vi "Main.vi"(7 "sweep rate, /min":dbl=0.2, 8 "sweep to:":dbl=-0.5, 9 "sweep":T6(radio)=enum."time_sweep") -> ()   [LabVIEW 2017] (continued)
                  n2525 = case shown="False" w3354 {
                    tunnel: w3355 -> [w3357 w3370]
                    tunnel: [w3357 w3369] -> w3356
                    frame False {
                      # "we are not measuring 2182A 4 channel 2 (2182A_4_ch2)"
                    }
                    frame True {
                      # "switching to channel 2 and then\nback to channel 1"
                      # "we are  measuring 2182A 4 channel 2 (2182A_4_ch2)"
                      n2526 = local read "2182A 4 addr"() -> (w3364:u8)
                      n2527 = Number To Decimal String(number=w3364) -> (decimal integer string=w3359:string)  [unwired: 1 in]
                      n2528 = GPIB Write(0:w3359, 1:":SENSe:CHAN 2") -> (6:w3361:errorcluster)  [unwired: 3 in, 1 out]
                      n2529 = GPIB Write(0:w3359, 1:":SENSe:DATA:FRES?", 3:w3361) -> (6:w3368:errorcluster)  [unwired: 2 in, 1 out]
                      n2530 = GPIB Read(0:w3359, 1:200, 3:w3368) -> (5:w3363:string, 7:w3360:errorcluster)  [unwired: 2 in, 1 out]
                      n2531 = GPIB Write(0:w3359, 1:":SENSe:CHAN 1", 3:w3360) -> ()  [unwired: 2 in, 2 out]
                      n2532 = Fract/Exp String To Number(string=w3363) -> (number=w3366:dbl)  [unwired: 3 in, 1 out]
                      n2533 = Build Array (concatenate)(w3370, w3366) -> (w3369:dbl[])
                    }
                  }
                  n2534 = property on="data" class="Arr (strict)"("Value"=w3356) -> ()  [unwired: 2 in, 2 out]
                }
                frame #34 {
                  # "check if voltage on\nKeithley 2636A smua\nis to be measured"
                  n2535 = local read "2636A smua meas v"() -> (w3371:bool)
                  n2536 = property on="data" class="Arr (strict)"() -> ("Value"=w3372:dbl[])  [unwired: 2 in, 2 out]
                  n2537 = case shown="True" w3371 {
                    tunnel: w3372 -> [w3374 w3380]
                    tunnel: [w3374 w3379] -> w3373
                    frame False {
                      # "we are not measuring voltage on 2636A smua (2636A_smua_v)"
                    }
                    frame True {
                      # "we are  measuring voltage on 2636A smua (2636A_smua_v)"
                      n2538 = local read "2336A addr"() -> (w3375:refnum<visa-resource-name>)
                      n2539 = call "SinglePointMeasurement.vi"("Measure"=Measure."Voltage", "Channel"=Channel."a", "VISA resource name 2"=w3375) -> ("Measuremet"=w3377:dbl)  [unwired: 3 in, 4 out]
                      n2540 = Build Array (concatenate)(w3380, w3377) -> (w3379:dbl[])
                    }
                  }
                  n2541 = property on="data" class="Arr (strict)"("Value"=w3373) -> ()  [unwired: 2 in, 2 out]
                }
                frame #35 {
                  # "check if current on\nKeithley 2636A smua\nis to be measured"
                  n2542 = local read "2636A smua meas i"() -> (w3381:bool)
                  n2543 = property on="data" class="Arr (strict)"() -> ("Value"=w3382:dbl[])  [unwired: 2 in, 2 out]
                  n2544 = case shown="True" w3381 {
                    tunnel: w3382 -> [w3384 w3387]
                    tunnel: [w3384 w3386] -> w3383
                    frame False {
                      # "we are not measuring current on 2636A smua (2636A_smua_i)"
                    }
                    frame True {
                      # "we are  measuring current on 2636A smua (2636A_smua_i)"
                      n2545 = stacked-sequence {
                        tunnel: [_ w3396] -> w3385
                        frame #0 {
                          n2546 = local read "auto\nrange A"() -> (w3391:bool)
                          n2547 = local read "2336A addr"() -> (w3394:refnum<visa-resource-name>)
                          n2548 = Select(t="smua.AUTORANGE_ON", s=w3391, f="smua.AUTORANGE_OFF") -> (s? t:f=w3389:string)
                          n2549 = Concatenate Strings("smua.measure.autorangei = ", w3389) -> (w3388:string)
                          n2550 = VISA Write(VISA resource name=w3394, write buffer=w3388) -> ()  [unwired: 1 in, 3 out]
                        }
                        frame #1 {
                          n2551 = local read "2336A addr"() -> (w3398:refnum<visa-resource-name>)
                          n2552 = call "SinglePointMeasurement.vi"("Measure"=Measure."Current", "Channel"=Channel."a", "VISA resource name 2"=w3398) -> ("Measuremet"=w3396:dbl)  [unwired: 3 in, 4 out]
                        }
                      }
                      n2553 = Build Array (concatenate)(w3387, w3385) -> (w3386:dbl[])
                    }
                  }
                  n2554 = property on="data" class="Arr (strict)"("Value"=w3383) -> ()  [unwired: 2 in, 2 out]
                }
                frame #36 {
                  # "check if voltage on\nKeithley 2636A smub\nis to be measured"
                  n2555 = local read "2636A smub meas v"() -> (w3399:bool)
                  n2556 = property on="data" class="Arr (strict)"() -> ("Value"=w3400:dbl[])  [unwired: 2 in, 2 out]
                  n2557 = case shown="True" w3399 {
                    tunnel: w3400 -> [w3402 w3408]
                    tunnel: [w3402 w3407] -> w3401
                    frame False {
                      # "we are not measuring voltage on 2636A smub (2636A_smub_v)"
                    }
                    frame True {
                      # "we are  measuring voltage on 2636A smub (2636A_smub_v)"
                      n2558 = local read "2336A addr"() -> (w3406:refnum<visa-resource-name>)
                      n2559 = call "SinglePointMeasurement.vi"("Measure"=Measure."Voltage", "Channel"=Channel."b", "VISA resource name 2"=w3406) -> ("Measuremet"=w3404:dbl)  [unwired: 3 in, 4 out]
                      n2560 = Build Array (concatenate)(w3408, w3404) -> (w3407:dbl[])
                    }
                  }
                  n2561 = property on="data" class="Arr (strict)"("Value"=w3401) -> ()  [unwired: 2 in, 2 out]
                }
                frame #37 {
                  # "check if current on\nKeithley 2636A smub\nis to be measured"
                  n2562 = local read "2636A smub meas i"() -> (w3409:bool)
                  n2563 = property on="data" class="Arr (strict)"() -> ("Value"=w3410:dbl[])  [unwired: 2 in, 2 out]
                  n2564 = case shown="True" w3409 {
                    tunnel: w3410 -> [w3412 w3415]
                    tunnel: [w3412 w3414] -> w3411
                    frame False {
                      # "we are not measuring current on 2636A smub (2636A_smub_i)"
                    }
                    frame True {
                      # "we are  measuring current on 2636A smub (2636A_smub_i)"
                      n2565 = stacked-sequence {
                        tunnel: [_ w3424] -> w3413
                        frame #0 {
                          n2566 = local read "auto\nrange B"() -> (w3419:bool)
                          n2567 = local read "2336A addr"() -> (w3422:refnum<visa-resource-name>)
                          n2568 = Select(t="smub.AUTORANGE_ON", s=w3419, f="smub.AUTORANGE_OFF") -> (s? t:f=w3417:string)
                          n2569 = Concatenate Strings("smub.measure.autorangei = ", w3417) -> (w3416:string)
                          n2570 = VISA Write(VISA resource name=w3422, write buffer=w3416) -> ()  [unwired: 1 in, 3 out]
                        }
                        frame #1 {
                          n2571 = local read "2336A addr"() -> (w3426:refnum<visa-resource-name>)
                          n2572 = call "SinglePointMeasurement.vi"("Measure"=Measure."Current", "Channel"=Channel."b", "VISA resource name 2"=w3426) -> ("Measuremet"=w3424:dbl)  [unwired: 3 in, 4 out]
                        }
                      }
                      n2573 = Build Array (concatenate)(w3415, w3413) -> (w3414:dbl[])
                    }
                  }
                  n2574 = property on="data" class="Arr (strict)"("Value"=w3411) -> ()  [unwired: 2 in, 2 out]
                }
                frame #38 {
                  # "check if time\nis to be measured"
                  n2575 = property on="data" class="Arr (strict)"() -> ("Value"=w3429:dbl[])  [unwired: 2 in, 2 out]
                  n2576 = local read "measure time"() -> (w3428:bool)
                  n2577 = case shown="True" w3428 {
                    tunnel: w3429 -> [w3431 w3437]
                    tunnel: [w3431 w3436] -> w3430
                    tunnel: w3427 -> [_ w3434]
                    frame False {
                      # "we are not measuring time"
                    }
                    frame True {
                      # "seconds from the beginning of month"
                      # "we are  measuring time"
                      n2578 = call "timeInSeconds.vi"() -> ("Numeric"=w3435:dbl, "current time"=w3432:timestamp)  [unwired: 2 in]
                      n2579 = property on="current time" class="AbsTime (strict)"("Value"=w3432) -> ()  [unwired: 2 in, 2 out]
                      n2580 = Subtract(x=w3435, y=w3434) -> (x-y=w3433:dbl)
                      n2581 = Build Array (concatenate)(w3437, w3433) -> (w3436:dbl[])
                    }
                  }
                  n2582 = property on="data" class="Arr (strict)"("Value"=w3430) -> ()  [unwired: 2 in, 2 out]
                }
                frame #39 {
                  n2583 = local read "iPS_MagnetField"() -> (w3438:bool)
                  n2584 = property on="data" class="Arr (strict)"() -> ("Value"=w3439:dbl[])  [unwired: 2 in, 2 out]
                  n2585 = case shown="True" w3438 {
                    tunnel: w3439 -> [w3441 w3446]
                    tunnel: [w3441 w3445] -> w3440
                    frame False {
                      # "we are not Measuring magnetic field on IPS120-0"
                    }
                    frame True {
                      # "Measure magnetic field on Teslatron_iPS_Field"
                      n2586 = local read "iPS_addr_sweep"() -> (w3444:refnum<visa-resource-name>)
                      n2587 = call "iPSread.vi"("iPSreadCtrl"=iPSreadCtrl."MagnetField", "VISA resource name"=w3444) -> ("number"=w3443:dbl)  [unwired: 6 in, 3 out]
                      n2588 = Build Array (concatenate)(w3446, w3443) -> (w3445:dbl[])
                    }
                  }
                  n2589 = property on="data" class="Arr (strict)"("Value"=w3440) -> ()  [unwired: 2 in, 2 out]
                }
                frame #40 {
                  n2590 = property on="data" class="Arr (strict)"() -> ("Value"=w3448:dbl[])  [unwired: 2 in, 2 out]
                  n2591 = property on="Magnet_T" class="Bool (strict)"() -> ("Value"=w3447:bool)  [unwired: 2 in, 2 out]
                  n2592 = case shown="True" w3447 {
                    tunnel: w3448 -> [w3450 w3455]
                    tunnel: [w3450 w3454] -> w3449
                    frame False {
                      # "we are not Measuring magnetic field on IPS120-0"
                    }
                    frame True {
                      # "Measure magnetic_T on Teslatron"
                      n2593 = local read "iPS_addr_sweep"() -> (w3453:refnum<visa-resource-name>)
                      n2594 = call "iPSread.vi"("iPSreadCtrl"=iPSreadCtrl."Magnet Temp", "VISA resource name"=w3453) -> ("number"=w3452:dbl)  [unwired: 6 in, 3 out]
                      n2595 = Build Array (concatenate)(w3455, w3452) -> (w3454:dbl[])
                    }
                  }
                  n2596 = property on="data" class="Arr (strict)"("Value"=w3449) -> ()  [unwired: 2 in, 2 out]
                }
                frame #41 {
                  n2597 = property on="data" class="Arr (strict)"() -> ("Value"=w3457:dbl[])  [unwired: 2 in, 2 out]
                  n2598 = property on="SH_T" class="Bool (strict)"() -> ("Value"=w3456:bool)  [unwired: 2 in, 2 out]
                  n2599 = case shown="True" w3456 {
                    tunnel: w3457 -> [w3459 w3464]
                    tunnel: [w3459 w3463] -> w3458
                    frame False {
                      # "we are not Measuring magnetic field on IPS120-0"
                    }
                    frame True {
                      # "Measure  SH_T on Teslatron"
                      n2600 = local read "iPS_addr_sweep"() -> (w3462:refnum<visa-resource-name>)
                      n2601 = call "iPSread.vi"("iPSreadCtrl"=iPSreadCtrl."Switch Heater Temp", "VISA resource name"=w3462) -> ("number"=w3461:dbl)  [unwired: 6 in, 3 out]
                      n2602 = Build Array (concatenate)(w3464, w3461) -> (w3463:dbl[])
                    }
                  }
                  n2603 = property on="data" class="Arr (strict)"("Value"=w3458) -> ()  [unwired: 2 in, 2 out]
                }
                frame #42 {
                  # "check if current \non 2461 SouceMeter\nis to be measured"
                  n2604 = property on="data" class="Arr (strict)"() -> ("Value"=w3466:dbl[])  [unwired: 2 in, 2 out]
                  n2605 = property on="iTC_Sample_T" class="Bool (strict)"() -> ("Value"=w3465:bool)  [unwired: 2 in, 2 out]
                  n2606 = case shown="True" w3465 {
                    tunnel: w3466 -> [w3468 w3473]
                    tunnel: [w3468 w3472] -> w3467
                    frame False {
                      # "we are not measuring 2461, voltage (2461_meas_v)"
                    }
                    frame True {
                      # "we are  measuring 2461, voltage (2461_meas_v)"
                      n2607 = property on="iTC_addr_sweep" class="VISAName"() -> ("Value"=w3471:refnum<visa-resource-name>)  [unwired: 2 in, 2 out]
                      n2608 = call "iTCread.vi"("VISA resource name"=w3471, "iTCreadCtrl"=iTCreadCtrl."Sample Temp") -> ("number"=w3469:dbl)  [unwired: 5 in, 3 out]
                      n2609 = Build Array (concatenate)(w3473, w3469) -> (w3472:dbl[])
                    }
                  }
                  n2610 = property on="data" class="Arr (strict)"("Value"=w3467) -> ()  [unwired: 2 in, 2 out]
                }
                frame #43 {
                  # "check if current \non 2461 SouceMeter\nis to be measured"
                  n2611 = property on="data" class="Arr (strict)"() -> ("Value"=w3475:dbl[])  [unwired: 2 in, 2 out]
                  n2612 = property on="VTI_T" class="Bool (strict)"() -> ("Value"=w3474:bool)  [unwired: 2 in, 2 out]
                  n2613 = case shown="True" w3474 {
                    tunnel: w3475 -> [w3477 w3482]
                    tunnel: [w3477 w3481] -> w3476
                    frame False {
                      # "we are not measuring 2461, voltage (2461_meas_v)"
                    }
                    frame True {
                      # "we are  measuring 2461, voltage (2461_meas_v)"
                      n2614 = property on="iTC_addr_sweep" class="VISAName"() -> ("Value"=w3480:refnum<visa-resource-name>)  [unwired: 2 in, 2 out]
                      n2615 = call "iTCread.vi"("VISA resource name"=w3480, "iTCreadCtrl"=iTCreadCtrl."VTI Temp") -> ("number"=w3478:dbl)  [unwired: 5 in, 3 out]
                      n2616 = Build Array (concatenate)(w3482, w3478) -> (w3481:dbl[])
                    }
                  }
                  n2617 = property on="data" class="Arr (strict)"("Value"=w3476) -> ()  [unwired: 2 in, 2 out]
                }
                frame #44 {
                  # "check if current \non 2461 SouceMeter\nis to be measured"
                  n2618 = property on="data" class="Arr (strict)"() -> ("Value"=w3484:dbl[])  [unwired: 2 in, 2 out]
                  n2619 = property on="PT1_T" class="Bool (strict)"() -> ("Value"=w3483:bool)  [unwired: 2 in, 2 out]
                  n2620 = case shown="True" w3483 {
                    tunnel: w3484 -> [w3486 w3491]
                    tunnel: [w3486 w3490] -> w3485
                    frame False {
                      # "we are not measuring 2461, voltage (2461_meas_v)"
                    }
                    frame True {
                      # "we are  measuring 2461, voltage (2461_meas_v)"
                      n2621 = property on="iTC_addr_sweep" class="VISAName"() -> ("Value"=w3489:refnum<visa-resource-name>)  [unwired: 2 in, 2 out]
                      n2622 = call "iTCread.vi"("VISA resource name"=w3489, "iTCreadCtrl"=iTCreadCtrl."PT1 Temp") -> ("number"=w3487:dbl)  [unwired: 5 in, 3 out]
                      n2623 = Build Array (concatenate)(w3491, w3487) -> (w3490:dbl[])
                    }
                  }
                  n2624 = property on="data" class="Arr (strict)"("Value"=w3485) -> ()  [unwired: 2 in, 2 out]
                }
                frame #45 {
                  # "check if current \non 2461 SouceMeter\nis to be measured"
                  n2625 = property on="data" class="Arr (strict)"() -> ("Value"=w3493:dbl[])  [unwired: 2 in, 2 out]
                  n2626 = property on="PT2_T" class="Bool (strict)"() -> ("Value"=w3492:bool)  [unwired: 2 in, 2 out]
                  n2627 = case shown="True" w3492 {
                    tunnel: w3493 -> [w3495 w3500]
                    tunnel: [w3495 w3499] -> w3494
                    frame False {
                      # "we are not measuring 2461, voltage (2461_meas_v)"
                    }
                    frame True {
                      # "we are  measuring 2461, voltage (2461_meas_v)"
                      n2628 = property on="iTC_addr_sweep" class="VISAName"() -> ("Value"=w3498:refnum<visa-resource-name>)  [unwired: 2 in, 2 out]
                      n2629 = call "iTCread.vi"("VISA resource name"=w3498, "iTCreadCtrl"=iTCreadCtrl."PT2 Temp") -> ("number"=w3496:dbl)  [unwired: 5 in, 3 out]
                      n2630 = Build Array (concatenate)(w3500, w3496) -> (w3499:dbl[])
                    }
                  }
                  n2631 = property on="data" class="Arr (strict)"("Value"=w3494) -> ()  [unwired: 2 in, 2 out]
                }
                frame #46 {
                  # "check if current \non 2461 SouceMeter\nis to be measured"
                  n2632 = property on="data" class="Arr (strict)"() -> ("Value"=w3502:dbl[])  [unwired: 2 in, 2 out]
                  n2633 = property on="VTI_P" class="Bool (strict)"() -> ("Value"=w3501:bool)  [unwired: 2 in, 2 out]
                  n2634 = case shown="True" w3501 {
                    tunnel: w3502 -> [w3504 w3509]
                    tunnel: [w3504 w3508] -> w3503
                    frame False {
                      # "we are not measuring 2461, voltage (2461_meas_v)"
                    }
                    frame True {
                      # "we are  measuring 2461, voltage (2461_meas_v)"
                      n2635 = property on="iTC_addr_sweep" class="VISAName"() -> ("Value"=w3507:refnum<visa-resource-name>)  [unwired: 2 in, 2 out]
                      n2636 = call "iTCread.vi"("VISA resource name"=w3507, "iTCreadCtrl"=iTCreadCtrl."VTI Pressure") -> ("number"=w3505:dbl)  [unwired: 5 in, 3 out]
                      n2637 = Build Array (concatenate)(w3509, w3505) -> (w3508:dbl[])
                    }
                  }
                  n2638 = property on="data" class="Arr (strict)"("Value"=w3503) -> ()  [unwired: 2 in, 2 out]
                }
                frame #47 {
                  # "check if current \non 2461 SouceMeter\nis to be measured"
                  n2639 = property on="2461_meas_v" class="Bool (strict)"() -> ("Value"=w3510:bool)  [unwired: 2 in, 2 out]
                  n2640 = property on="data" class="Arr (strict)"() -> ("Value"=w3511:dbl[])  [unwired: 2 in, 2 out]
                  n2641 = case shown="True" w3510 {
                    tunnel: w3511 -> [w3513 w3518]
                    tunnel: [w3513 w3517] -> w3512
                    frame False {
                      # "we are not measuring 2461, voltage (2461_meas_v)"
                    }
                    frame True {
                      # "we are  measuring 2461, voltage (2461_meas_v)"
                      n2642 = property on="2461_addr_sweep" class="VISAName"() -> ("Value"=w3515:refnum<visa-resource-name>)  [unwired: 2 in, 2 out]
                      n2643 = call <instrlib>:"Read (Single Point).vi"("VISA resource name"=w3515) -> ("Data out"=w3514:string)  [unwired: 12 in, 2 out]
                      n2644 = Fract/Exp String To Number(string=w3514) -> (number=w3516:dbl)  [unwired: 3 in, 1 out]
                      n2645 = Build Array (concatenate)(w3518, w3516) -> (w3517:dbl[])
                    }
                  }
                  n2646 = property on="data" class="Arr (strict)"("Value"=w3512) -> ()  [unwired: 2 in, 2 out]
                }
                frame #48 {
                  # "check if current \non 2461 SouceMeter\nis to be measured"
                  n2647 = property on="2461_meas_i" class="Bool (strict)"() -> ("Value"=w3519:bool)  [unwired: 2 in, 2 out]
                  n2648 = property on="data" class="Arr (strict)"() -> ("Value"=w3520:dbl[])  [unwired: 2 in, 2 out]
                  n2649 = case shown="True" w3519 {
                    tunnel: w3520 -> [w3522 w3526]
                    tunnel: [w3522 w3525] -> w3521
                    frame False {
                      # "we are not measuring 2461, voltage (2461_meas_v)"
                    }
                    frame True {
                      # "we are  measuring 2461, curent (2461_meas_i)"
                      n2650 = property on="2461_addr_sweep" class="VISAName"() -> ("Value"=w3524:refnum<visa-resource-name>)  [unwired: 2 in, 2 out]
                      n2651 = call <instrlib>:"Get Source Level.vi"("VISA resource name"=w3524) -> ("Current Level Out"=w3523:dbl)  [unwired: 7 in, 3 out]
                      n2652 = Build Array (concatenate)(w3526, w3523) -> (w3525:dbl[])
                    }
                  }
                  n2653 = property on="data" class="Arr (strict)"("Value"=w3521) -> ()  [unwired: 2 in, 2 out]
                }
                frame #49 {
                  # "Record Step Value \nif it is mapping"
                  n2654 = property on="Step Loop" class="Bool (strict)"() -> ("Value"=w3528:bool)  [unwired: 2 in, 2 out]
                  n2655 = property on="data" class="Arr (strict)"() -> ("Value"=w3529:dbl[])  [unwired: 2 in, 2 out]
                  n2656 = case shown="True" w3528 {
                    tunnel: w3529 -> [w3530 w3533]
                    tunnel: [w3530 w3532] -> w3527
                    frame False {
                      # "We are not recording Step Value if it is linetrace"
                    }
                    frame True {
                      # "We are recording Step Value if it is mapping"
                      n2657 = property on="Current Step Value" class="DigNum (strict)"() -> ("Value"=w3531:dbl)  [unwired: 2 in, 2 out]
                      n2658 = Build Array (concatenate)(w3533, w3531) -> (w3532:dbl[])
                    }
                  }
                  n2659 = property on="data" class="Arr (strict)"("Value"=w3527) -> ()  [unwired: 2 in, 2 out]
                }
                frame #50 {
                  # "Record Step Value \nif it is mapping"
                  n2660 = property on="HyperLoop" class="Bool (strict)"() -> ("Value"=w3534:bool)  [unwired: 2 in, 2 out]
                  n2661 = property on="data" class="Arr (strict)"() -> ("Value"=w3536:dbl[])  [unwired: 2 in, 2 out]
                  n2662 = case shown="True" w3534 {
                    tunnel: w3536 -> [w3537 w3540]
                    tunnel: [w3537 w3539] -> w3535
                    frame False {
                      # "We are not recording Step Value if it is linetrace"
                    }
                    frame True {
                      # "We are recording Step Value if it is mapping"
                      n2663 = property on="Current Hyper Value" class="DigNum (strict)"() -> ("Value"=w3538:dbl)  [unwired: 2 in, 2 out]
                      n2664 = Build Array (concatenate)(w3540, w3538) -> (w3539:dbl[])
                    }
                  }
                  n2665 = property on="data" class="Arr (strict)"("Value"=w3535) -> ()  [unwired: 2 in, 2 out]
                }
                frame #51 {
                  # "Record Step Value \nif it is mapping"
                  n2666 = property on="SuperHyper" class="Bool (strict)"() -> ("Value"=w3541:bool)  [unwired: 2 in, 2 out]
                  n2667 = property on="data" class="Arr (strict)"() -> ("Value"=w3543:dbl[])  [unwired: 2 in, 2 out]
                  n2668 = case shown="True" w3541 {
                    tunnel: w3543 -> [w3544 w3547]
                    tunnel: [w3544 w3546] -> w3542
                    frame False {
                      # "We are not recording Step Value if it is linetrace"
                    }
                    frame True {
                      # "We are recording SuperHyper_step if it is mapping"
                      n2669 = property on="Current SuperHyper Value" class="DigNum (strict)"() -> ("Value"=w3545:dbl)  [unwired: 2 in, 2 out]
                      n2670 = Build Array (concatenate)(w3547, w3545) -> (w3546:dbl[])
                    }
                  }
                  n2671 = property on="data" class="Arr (strict)"("Value"=w3542) -> ()  [unwired: 2 in, 2 out]
                }
              }
            }
            frame #4 {
              # "this part appends last\nmeasured point to the \ndata file"
              n2672 = local read "Data file:"() -> (w3549:path)
              n2673 = property on="data" class="Arr (strict)"() -> ("Value"=w3548:dbl[])  [unwired: 2 in, 2 out]
              n2674 = call-poly <vilib>:"Write To Spreadsheet File.vi"("format (%.3f)"="%.6e", "append to file? (new file:F)"=TRUE, "1D data"=w3548, "file path (dialog if empty)"=w3549) -> ()  [unwired: 4 in, 1 out]
            }
            frame #5 {
              n2675 = property on="data" class="Arr (strict)"() -> ("Value"=w3552:dbl[])  [unwired: 2 in, 2 out]
            }
          }
          n2676 = stacked-sequence "add data to array" {
            tunnel: w2845 -> [w3683]
            tunnel: [w3682] -> w2844
            tunnel: w2831 -> [w3681]
            frame #0 {
              n2677 = Build Array (concatenate)(w3683, w3681) -> (w3682:dbl[][])
            }
          }
          n2678 = And(x=w2833, y="Continuous Sweep") -> (x .and. y?=w2837:bool)
          n2679 = case shown="True" w2837 {
            frame False {
            }
            frame True {
              n2680 = property on="upper limit" class="DigNum (strict)"() -> ("Value"=w2846:dbl)  [unwired: 2 in, 2 out]
              n2681 = local read "sweep to:"() -> (w2848:dbl)
              n2682 = property on="lower limit" class="DigNum (strict)"() -> ("Value"=w2847:dbl)  [unwired: 2 in, 2 out]
              n2683 = Equal?(x=w2848, y=w2846) -> (x = y?=w2849:bool)
              n2684 = Select(t=w2847, s=w2849, f=w2846) -> (s? t:f=w2850:dbl)
              n2685 = local write "sweep to:"(w2850) -> ()
            }
          }
          n2686 = stacked-sequence "plot selected measurements" {
            seq-local: [_ w3706 _] -> [_ _ w3751]
            seq-local: [_ w3705 _] -> [_ _ w3752]
            tunnel: w2844 -> [_ w3704 _]
            frame #0 {
              n2687 = property on="XY Graph" class="XYGraph (strict)"("ActYScl"=0 ("Active Y Scale")) -> (error out=w3689:errorcluster)  [unwired: 2 in, 1 out]
              n2688 = property on="Show cursor" class="Bool (strict)"() -> ("Value"=w3684:bool)  [unwired: 2 in, 2 out]
              n2689 = property on="Xaxis" class="Ring (strict)"() -> ("Value"=w3694:u16)  [unwired: 2 in, 2 out]
              n2690 = property on="Yaxis" class="Ring (strict)"(error in=w3689) -> (error out=w3688:errorcluster, "RingText.Text"=w3687:string)  [unwired: 1 in, 1 out]
              n2691 = property on="XY Graph" class="XYGraph (strict)"("Cursor.Visible"=w3684) -> ()  [unwired: 2 in, 2 out]
              n2692 = property on="Figure_axis" class="Arr (strict)"() -> ("Value"=w3695:string[])  [unwired: 2 in, 2 out]
              n2693 = property on="XY Graph" class="XYGraph (strict)"(error in=w3688, "YScale.NameLbl.Text"=w3687) -> (error out=w3685:errorcluster)  [unwired: 1 in, 1 out]
              n2694 = property on="XY Graph" class="XYGraph (strict)"(error in=w3685, "ActYScl"=1 ("Active Y Scale")) -> (error out=w3691:errorcluster)  [unwired: 1 in, 1 out]
              n2695 = property on="Yright" class="Ring (strict)"(error in=w3691) -> (error out=w3692:errorcluster, "RingText.Text"=w3686:string)  [unwired: 1 in, 1 out]
              n2696 = Index Array(array=w3695, index=w3694) -> (element=w3696:string)
              n2697 = property on="XY Graph" class="XYGraph (strict)"("XScale.NameLbl.Text"=w3696) -> ()  [unwired: 2 in, 2 out]
              n2698 = property on="XY Graph" class="XYGraph (strict)"(error in=w3692, "YScale.NameLbl.Text"=w3686) -> ()  [unwired: 1 in, 2 out]
            }
            frame #1 {
              n2699 = local read "Xaxis"() -> (w3709:u16)
              n2700 = property on="Yright" class="Ring (strict)"() -> ("Value"=w3703:u16)  [unwired: 2 in, 2 out]
              n2701 = property on="Yright" class="Ring (strict)"() -> ("RingText.Text"=w3702:string)  [unwired: 2 in, 2 out]
              n2702 = property on="Xaxis" class="Ring (strict)"() -> ("RingText.Text"=w3708:string)  [unwired: 2 in, 2 out]
              n2703 = property on="Yaxis" class="Ring (strict)"() -> ("RingText.Text"=w3707:string)  [unwired: 2 in, 2 out]
              n2704 = local read "Yaxis"() -> (w3710:u16)
              n2705 = case shown="\"formula\"" w3702 {
                tunnel: [w3715 w3722] -> w3700
                tunnel: w3703 -> [_ w3721]
                tunnel: w3704 -> [w3716 w3720]
                tunnel: [w3714 errorcluster {"status"=FALSE, "code"=0, "source"=""} ("error out")] -> _
                frame "formula" {
                  n2706 = local read "formula_variables"() -> (w3717:string[])
                  n2707 = Transpose 2D Array(2D array=w3716) -> (transposed array=w3718:dbl[][])
                  n2708 = property on="Y_right_formula" class="Str"() -> ("Value"=w3713:string)  [unwired: 2 in, 2 out]
                  n2709 = call <vilib>:"Eval Multi-Variable Array.vi"("Variables"=w3717, "X Values"=w3718, "formula"=w3713) -> ("error out"=w3714:errorcluster, "Y Values"=w3715:dbl[])  [unwired: 1 in]
                }
                frame "0", Default {
                  n2710 = Index Array(array=w3720, index (col)=w3721) -> (element=w3722:dbl[])  [unwired: 1 in]
                }
              }
              n2711 = case shown="\"formula\"" w3708 {
                tunnel: [w3733 w3738] -> w3712
                tunnel: w3709 -> [w3736 _]
                tunnel: w3704 -> [w3735 w3742]
                tunnel: [errorcluster {"status"=FALSE, "code"=0, "source"=""} ("error out") w3739] -> w3706
                tunnel: [w3733 w3738] -> w3701
                frame "0", Default {
                  n2712 = Index Array(array=w3735, index (col)=w3736) -> (element=w3733:dbl[])  [unwired: 1 in]
                }
                frame "formula" {
                  n2713 = local read "formula_variables"() -> (w3741:string[])
                  n2714 = Transpose 2D Array(2D array=w3742) -> (transposed array=w3740:dbl[][])
                  n2715 = property on="X_axis_formula" class="Str"() -> ("Value"=w3737:string)  [unwired: 2 in, 2 out]
                  n2716 = call <vilib>:"Eval Multi-Variable Array.vi"("Variables"=w3741, "X Values"=w3740, "formula"=w3737) -> ("error out"=w3739:errorcluster, "Y Values"=w3738:dbl[])  [unwired: 1 in]
                }
              }
              n2717 = case shown="\"formula\"" w3707 {
                tunnel: [w3725 w3732] -> w3711
                tunnel: w3710 -> [_ w3731]
                tunnel: w3704 -> [w3726 w3730]
                tunnel: [w3724 errorcluster {"status"=FALSE, "code"=0, "source"=""} ("error out")] -> w3705
                frame "formula" {
                  n2718 = local read "formula_variables"() -> (w3727:string[])
                  n2719 = Transpose 2D Array(2D array=w3726) -> (transposed array=w3728:dbl[][])
                  n2720 = property on="Y_left_formula" class="Str"() -> ("Value"=w3723:string)  [unwired: 2 in, 2 out]
                  n2721 = call <vilib>:"Eval Multi-Variable Array.vi"("Variables"=w3727, "X Values"=w3728, "formula"=w3723) -> ("error out"=w3724:errorcluster, "Y Values"=w3725:dbl[])  [unwired: 1 in]
                }
                frame "0", Default {
                  n2722 = Index Array(array=w3730, index (col)=w3731) -> (element=w3732:dbl[])  [unwired: 1 in]
                }
              }
              n2723 = Bundle("Y Values"=w3712, "Y Values"=w3711) -> (w3699:cluster{"Y Values":dbl[], "Y Values":dbl[]})  [unwired: 1 in]
              n2724 = Bundle("Y Values"=w3701, "Y Values"=w3700) -> (w3698:cluster{"Y Values":dbl[], "Y Values":dbl[]})  [unwired: 1 in]
              n2725 = Build Array(w3699, w3698) -> (w3697:cluster{"Y Values":dbl[], "Y Values":dbl[]}[])
              n2726 = property on="XY Graph" class="XYGraph (strict)"("Value"=w3697) -> ()  [unwired: 2 in, 2 out]
            }
            frame #2 {
              # "show if formula \nis wrong"
              n2727 = property on="Yaxis" class="Ring (strict)"() -> ("RingText.Text"=w3748:string)  [unwired: 2 in, 2 out]
              n2728 = property on="XY Graph" class="XYGraph (strict)"("Active Plot"=u32 0, "Plot.Plot Name"=w3748) -> (error out=w3749:errorcluster)  [unwired: 2 in, 1 out]
              n2729 = property on="Yright" class="Ring (strict)"() -> ("RingText.Text"=w3746:string)  [unwired: 2 in, 2 out]
              n2730 = property on="XY Graph" class="XYGraph (strict)"(error in=w3749, "Active Plot"=u32 1, "Plot.Plot Name"=w3746) -> ()  [unwired: 1 in, 2 out]
              n2731 = Unbundle By Name(w3752) -> ("status"=w3745:bool)
              n2732 = Unbundle By Name(w3751) -> ("status"=w3744:bool)
              n2733 = Unbundle By Name(w3751) -> ("status"=w3743:bool)
              n2734 = property on="status 3" class="Bool (strict)"("Value"=w3743) -> ()  [unwired: 2 in, 2 out]
              n2735 = property on="status 2" class="Bool (strict)"("Value"=w3745) -> ()  [unwired: 2 in, 2 out]
              n2736 = property on="status" class="Bool (strict)"("Value"=w3744) -> ()  [unwired: 2 in, 2 out]
            }
          }
          n2737 = stacked-sequence "set next value in the sweep" {
            tunnel: w2843 -> [w3558 _]
            tunnel: [w3558 _] -> w2842
            tunnel: w2840 -> [_ w3676]
            tunnel: w2835 -> [w3561 _]
            frame #0 {
              n2738 = local read "sweep"() -> (w3564:T6)
              n2739 = property on="Sweep Channel" class="DigNum (strict)"("Value"=w3558) -> ()  [unwired: 2 in, 2 out]
              n2740 = property on="sweep value" class="DigNum (strict)"("Value"=w3558) -> ()  [unwired: 2 in, 2 out]
              n2741 = case shown="\"iPS\"" w3564 {
                tunnel: w3558 -> [w3577 w3585 w3591 w3600 w3622 _ w3624 w3647 w3671]
                tunnel: w3561 -> [_ _ _ w3598 _ _ _ _ _]
                frame "2400_1" {
                  # "sweep voltage on 2400 1"
                  n2742 = local read "2400 1 addr"() -> (w3579:u8)
                  n2743 = Number To Fractional String(number=w3577) -> (F-format string=w3583:string)  [unwired: 3 in]
                  n2744 = Concatenate Strings(":INIT:IMM; :SOUR:VOLT:LEV:IMM:AMPL " ("data"), w3583) -> (w3581:string)
                  n2745 = Number To Decimal String(number=w3579) -> (decimal integer string=w3578:string)  [unwired: 1 in]
                  n2746 = GPIB Write(0:w3578, 1:w3581, 2:i16 1 ("mode (0)")) -> ()  [unwired: 2 in, 2 out]
                }
                frame "2400_2" {
                  # "sweep curr on 2400 2"
                  n2747 = Number To Fractional String(number=w3585) -> (F-format string=w3590:string)  [unwired: 3 in]
                  n2748 = local read "2400 2 addr"() -> (w3587:u8)
                  n2749 = Concatenate Strings(":INIT:IMM; :SOUR:CURR:LEV:IMM:AMPL " ("data"), w3590) -> (w3588:string)
                  n2750 = Number To Decimal String(number=w3587) -> (decimal integer string=w3586:string)  [unwired: 1 in]
                  n2751 = GPIB Write(0:w3586, 1:w3588, 2:i16 1 ("mode (0)")) -> ()  [unwired: 2 in, 2 out]
                }
                frame "2400_3" {
                  # "sweep voltage on 2400 3"
                  n2752 = local read "2400 3 addr"() -> (w3593:u8)
                  n2753 = Number To Fractional String(number=w3591) -> (F-format string=w3597:string)  [unwired: 3 in]
                  n2754 = Concatenate Strings(":INIT:IMM; :SOUR:VOLT:LEV:IMM:AMPL " ("data"), w3597) -> (w3595:string)
                  n2755 = Number To Decimal String(number=w3593) -> (decimal integer string=w3592:string)  [unwired: 1 in]
                  n2756 = GPIB Write(0:w3592, 1:w3595, 2:i16 1 ("mode (0)")) -> ()  [unwired: 2 in, 2 out]
                }
                frame "2636a_smua" {
                  n2757 = case shown="False" "sweep 2" {
                    tunnel: w3600 -> [w3605 w3618]
                    tunnel: w3598 -> [w3602 _]
                    frame True {
                      w3603 = 30.0 ("y")
                      n2758 = Subtract(x=w3605, y=w3602) -> (x-y=w3604:dbl)
                      n2759 = Divide(x=w3604, y=w3603) -> (x/y=w3601:dbl)
                      n2760 = for {
                        N: w3603 -> [_]
                        tunnel: w3602 -> [w3611]
                        tunnel: w3601 -> [w3609]
                        i -> [w3610]
                        n2761 = Multiply(x=w3609, y=w3610) -> (x*y=w3608:dbl)
                        n2762 = local read "2336A addr"() -> (w3613:refnum<visa-resource-name>)
                        n2763 = Add(x=w3608, y=w3611) -> (x+y=w3607:dbl)
                        n2764 = call "setLevel.vi"("VISA resource name 2"=w3613, "Source"=Source."Voltage", "Channel"=Channel."a", "SourceLevel"=w3607) -> ()  [unwired: 1 in, 3 out]
                        n2765 = Wait (ms)(milliseconds to wait=u32 12) -> ()  [unwired: 1 out]
                      }
                    }
                    frame False {
                      # "sweep voltage on 2636a smua"
                      n2766 = local read "2336A addr"() -> (w3616:refnum<visa-resource-name>)
                      n2767 = call "setLevel.vi"("VISA resource name 2"=w3616, "Source"=Source."Voltage", "Channel"=Channel."a", "SourceLevel"=w3618) -> ()  [unwired: 1 in, 3 out]
                    }
                  }
                }
                frame "2636a_smub" {
                  # "sweep voltage on 2636b smua"
                  n2768 = local read "2336A addr"() -> (w3619:refnum<visa-resource-name>)
                  n2769 = call "setLevel.vi"("VISA resource name 2"=w3619, "Source"=Source."Voltage", "Channel"=Channel."b", "SourceLevel"=w3622) -> ()  [unwired: 1 in, 3 out]
                }
                frame "time_sweep", Default {
                  # "do not sweep, just time"
                }
                frame "iPS" {
                  n2770 = property on="Sweep B" class="Bool (strict)"() -> ("Value"=w3623:bool)  [unwired: 2 in, 2 out]
                  n2771 = case shown="True" w3623 {
                    tunnel: w3624 -> [_ w3625]
                    frame False {
                      # "Time as dummy B field"
                    }
                    frame True {
                      n2772 = stacked-sequence {
                        tunnel: w3625 -> [w3628 _ w3636 w3638]
                        frame #0 {
                          n2773 = local read "iPS_addr_sweep"() -> (w3627:refnum<visa-resource-name>)
                          n2774 = call "iPSset.vi"("Target Field, T"=w3628, "iPSSetCtrl"=iPSsetCtrl."Set Target Field", "VISA resource name"=w3627) -> ()  [unwired: 5 in, 4 out]
                        }
                        frame #1 {
                          n2775 = local read "iPS_addr_sweep"() -> (w3631:refnum<visa-resource-name>)
                          n2776 = property on="sweep rate, /min" class="DigNum (strict)"() -> ("Value"=w3629:dbl)  [unwired: 2 in, 2 out]
                          n2777 = call "iPSset.vi"("Field Rate, T/min"=w3629, "iPSSetCtrl"=iPSsetCtrl."Set Target Field Rate", "VISA resource name"=w3631) -> ()  [unwired: 5 in, 4 out]
                        }
                        frame #2 {
                          n2778 = Not Equal To 0?(x=w3636) -> (x != 0?=w3634:bool)
                          n2779 = local read "iPS_addr_sweep"() -> (w3637:refnum<visa-resource-name>)
                          n2780 = Select(t=iPSsetCtrl."Go to Field" ("iPSSetCtrl"), s=w3634, f=iPSsetCtrl."Go to Field" ("iPSSetCtrl")) -> (s? t:f=w3632:T18)
                          n2781 = call "iPSset.vi"("iPSSetCtrl"=w3632, "VISA resource name"=w3637) -> ()  [unwired: 6 in, 4 out]
                        }
                        frame #3 {
                          n2782 = while {
                            tunnel: w3638 -> [w3641]
                            stop <- w3644 stop-if-true
                            n2783 = property on="iPS_addr_sweep" class="VISAName"() -> ("Value"=w3640:refnum<visa-resource-name>)  [unwired: 2 in, 2 out]
                            n2784 = call "iPSread.vi"("iPSreadCtrl"=iPSreadCtrl."MagnetField", "VISA resource name"=w3640) -> ("number"=w3643:dbl)  [unwired: 6 in, 3 out]
                            n2785 = property on="Tolerance_Sweep" class="DigNum (strict)"() -> ("Value"=w3642:dbl)  [unwired: 2 in, 2 out]
                            n2786 = Subtract(x=w3643, y=w3641) -> (x-y=w3646:dbl)
                            n2787 = Absolute Value(x=w3646) -> (abs(x)=w3645:dbl)
                            n2788 = Less Or Equal?(x=w3645, y=w3642) -> (x <= y?=w3644:bool)
                          }
                        }
                      }
                    }
                  }
                }
                frame "iTC" {
                  n2789 = stacked-sequence {
                    tunnel: w3647 -> [w3649 w3656 w3661]
                    frame #0 {
                      n2790 = Decrement(x=w3649) -> (x-1=w3651:dbl)
                      n2791 = property on="iTC_addr_sweep" class="VISAName"() -> ("Value"=w3648:refnum<visa-resource-name>)  [unwired: 2 in, 2 out]
                      n2792 = Less Or Equal To 0?(x=w3651) -> (x <= 0?=w3653:bool)
                      n2793 = Select(t=0.0, s=w3653, f=w3651) -> (s? t:f=w3650:dbl)
                      n2794 = call "iTCset.vi"("Set Point"=w3650, "iTCSetCtrl"=iTCsetCtrl."Set VTI Temp", "VISA resource name"=w3648) -> ()  [unwired: 5 in, 4 out]
                    }
                    frame #1 {
                      n2795 = Less Or Equal To 0?(x=w3656) -> (x <= 0?=w3659:bool)
                      n2796 = property on="iTC_addr_sweep" class="VISAName"() -> ("Value"=w3655:refnum<visa-resource-name>)  [unwired: 2 in, 2 out]
                      n2797 = Select(t=0.0, s=w3659, f=w3656) -> (s? t:f=w3657:dbl)
                      n2798 = call "iTCset.vi"("Set Point"=w3657, "iTCSetCtrl"=iTCsetCtrl."Set Sample Temp", "VISA resource name"=w3655) -> ()  [unwired: 5 in, 4 out]
                    }
                    frame #2 {
                      n2799 = disable-structure shown="Disabled" {
                        disable-tunnel: w3661 -> [w3662 _]
                        frame Disabled {
                          n2800 = while {
                            tunnel: w3662 -> [w3665]
                            stop <- w3666 stop-if-true
                            n2801 = property on="iTC_addr_sweep" class="VISAName"() -> ("Value"=w3663:refnum<visa-resource-name>)  [unwired: 2 in, 2 out]
                            n2802 = call "iTCread.vi"("iTCreadCtrl"=iTCreadCtrl."Sample Temp", "VISA resource name"=w3663) -> ("number"=w3669:dbl)  [unwired: 6 in, 3 out]
                            n2803 = Subtract(x=w3669, y=w3665) -> (x-y=w3668:dbl)
                            n2804 = property on="Tolerance_Sweep" class="DigNum (strict)"() -> ("Value"=w3664:dbl)  [unwired: 2 in, 2 out]
                            n2805 = Absolute Value(x=w3668) -> (abs(x)=w3667:dbl)
                            n2806 = Less?(x=w3667, y=w3664) -> (x < y?=w3666:bool)
                          }
                        }
                        frame Enabled {
                        }
                      }
                    }
                  }
                }
                frame "2461" {
                  w3672 = u16 1 items=["Volts", "Current"] ("Function (0: Volts)")
                  n2807 = property on="2461_addr_sweep" class="VISAName"() -> ("Value"=w3673:refnum<visa-resource-name>)  [unwired: 2 in, 2 out]
                  n2808 = call <instrlib>:"Configure Source Level.vi"("Source Level (1.0)"=w3671, "Function (0: Volts)"=w3672, "VISA resource name"=w3673) -> ()  [unwired: 7 in, 2 out]
                }
              }
              n2809 = property on="Slope" class="DigNum (strict)"() -> ("Value"=w3559:dbl)  [unwired: 2 in, 2 out]
              n2810 = property on="Offset" class="DigNum (strict)"() -> ("Value"=w3560:dbl)  [unwired: 2 in, 2 out]
              n2811 = Multiply(x=w3559, y=w3558) -> (x*y=w3562:dbl)
              n2812 = local read "sweep"() -> (w3556:T6)
              n2813 = property on="Double Sweep" class="Bool (strict)"() -> ("Value"=w3555:bool)  [unwired: 2 in, 2 out]
              n2814 = Add(x=w3560, y=w3562) -> (x+y=w3563:dbl)
              n2815 = property on="Lead Chanl" class="Enum (strict)"() -> ("Value"=w3557:T1)  [unwired: 2 in, 2 out]
              n2816 = Equal?(x=w3556, y=w3557) -> (x = y?=w3554:bool)
              n2817 = And(x=w3555, y=w3554) -> (x .and. y?=w3553:bool)
              n2818 = case shown="True" w3553 {
                tunnel: w3563 -> [_ w3565]
                frame False {
                }
                frame True {
                  n2819 = disable-structure shown="Enabled" {
                    disable-tunnel: w3565 -> [w3566 w3574]
                    frame Disabled {
                      # "sweep voltage on 2400 2"
                      n2820 = local read "2400 2 addr"() -> (w3567:u8)
                      n2821 = Number To Fractional String(number=w3566) -> (F-format string=w3568:string)  [unwired: 3 in]
                      n2822 = Concatenate Strings(":INIT:IMM; :SOUR:VOLT:LEV:IMM:AMPL " ("data"), w3568) -> (w3570:string)
                      n2823 = Number To Decimal String(number=w3567) -> (decimal integer string=w3571:string)  [unwired: 1 in]
                      n2824 = GPIB Write(0:w3571, 1:w3570, 2:i16 1 ("mode (0)")) -> ()  [unwired: 2 in, 2 out]
                    }
                    frame Enabled {
                      n2825 = property on="Slave Channel" class="Enum (strict)"() -> ("Value"=w3573:T2)  [unwired: 2 in, 2 out]
                      n2826 = local read "2336A addr"() -> (w3576:refnum<visa-resource-name>)
                      n2827 = call "setLevel.vi"("VISA resource name 2"=w3576, "Source"=Source."Voltage", "Channel"=w3573, "SourceLevel"=w3574) -> ()  [unwired: 1 in, 3 out]
                    }
                  }
                }
              }
            }
            frame #1 {
              # "calculate deliberate time delay for the next step"
              n2828 = Tick Count (ms)() -> (millisecond timer value=w3678:u32)
              n2829 = Subtract(x=w3678, y=w3676) -> (x-y=w3677:u32)
              n2830 = property on="time/point, sec" class="DigNum (strict)"() -> ("Value"=w3679:dbl)  [unwired: 2 in, 2 out]
              n2831 = Multiply(x=w3679, y=1000.0) -> (x*y=w3675:dbl)
              n2832 = Subtract(x=w3675, y=w3677) -> (x-y=w3674:dbl)
              n2833 = property on="time delay, ms" class="DigNum (strict)"("Value"=w3674) -> ()  [unwired: 2 in, 2 out]
            }
          }
          n2834 = Not(x="Continuous Sweep") -> (.not. x?=w2836:bool)
          n2835 = And(x=w2833, y=w2836) -> (x .and. y?=w2834:bool)
          n2836 = Or(x=w2834, y="Stop Sweep") -> (x .or. y?=w2832:bool)
        }
        n2837 = stacked-sequence {
          tunnel: w1796 -> [_ _ _]
          tunnel: w1795 -> [_ _ w2808]
          frame #0 {
            n2838 = property on="Step Loop" class="Bool (strict)"() -> ("Value"=w2794:bool)  [unwired: 2 in, 2 out]
            n2839 = case shown="False" w2794 {
              frame False {
                w2796 = T12."Enabled" ("Disabled")
                w2795 = T12."Enabled" ("Disabled")
                # "Return the buttons to Idle state"
                n2840 = property on="sweep" class="RadioBtnsControl (strict)"("DisabledEnum"=w2795) -> ()  [unwired: 2 in, 2 out]
                n2841 = property on="2182A 1 addr" class="DigNum (strict)"("DisabledEnum"=w2795) -> ()  [unwired: 2 in, 2 out]
                n2842 = property on="2182A 2 addr" class="DigNum (strict)"("DisabledEnum"=w2795) -> ()  [unwired: 2 in, 2 out]
                n2843 = property on="2182A 3 addr" class="DigNum (strict)"("DisabledEnum"=w2795) -> ()  [unwired: 2 in, 2 out]
                n2844 = property on="2182A 4 addr" class="DigNum (strict)"("DisabledEnum"=w2795) -> ()  [unwired: 2 in, 2 out]
                n2845 = property on="2400 1 addr" class="DigNum (strict)"("DisabledEnum"=w2795) -> ()  [unwired: 2 in, 2 out]
                n2846 = property on="2400 2 addr" class="DigNum (strict)"("DisabledEnum"=w2795) -> ()  [unwired: 2 in, 2 out]
                n2847 = property on="2400 3 addr" class="DigNum (strict)"("DisabledEnum"=w2795) -> ()  [unwired: 2 in, 2 out]
                n2848 = property on="2336A addr" class="VISAName"("DisabledEnum"=w2795) -> ()  [unwired: 2 in, 2 out]
                n2849 = property on="SR830 1 addr" class="DigNum (strict)"("DisabledEnum"=w2795) -> ()  [unwired: 2 in, 2 out]
                n2850 = property on="SR830 2 addr" class="DigNum (strict)"("DisabledEnum"=w2795) -> ()  [unwired: 2 in, 2 out]
                n2851 = property on="SR830 3 addr" class="DigNum (strict)"("DisabledEnum"=w2795) -> ()  [unwired: 2 in, 2 out]
                n2852 = property on="SR830 4 addr" class="DigNum (strict)"("DisabledEnum"=w2795) -> ()  [unwired: 2 in, 2 out]
                n2853 = property on="sweep to:" class="DigNum (strict)"("DisabledEnum"=w2796) -> ()  [unwired: 2 in, 2 out]
                n2854 = property on="sweep rate, /min" class="DigNum (strict)"("DisabledEnum"=w2796) -> ()  [unwired: 2 in, 2 out]
              }
              frame True {
              }
            }
            n2855 = property on="Stop Sweep" class="Bool"("DisabledEnum"=T12."Disabled and Grayed Out" ("Disabled")) -> ()  [unwired: 2 in, 2 out]
          }
          frame #1 {
            n2856 = stacked-sequence {
              frame #0 {
                n2857 = local read "sweep"() -> (w2799:T6)
                n2858 = Equal?(x=w2799, y=T19."Radio Selection 7" ("sweep")) -> (x = y?=w2797:bool)
                n2859 = case shown="True" w2797 {
                  frame False {
                  }
                  frame True {
                    n2860 = local read "iPS_addr_sweep"() -> (w2800:refnum<visa-resource-name>)
                    n2861 = call "iPSset.vi"("iPSSetCtrl"=iPSsetCtrl."Hold", "VISA resource name"=w2800) -> ()  [unwired: 6 in, 4 out]
                  }
                }
              }
              frame #1 {
                n2862 = local read "2636A smua meas v"() -> (w2806:bool)
                n2863 = local read "2636A smub meas v"() -> (w2804:bool)
                n2864 = local read "2636A smub meas i"() -> (w2803:bool)
                n2865 = local read "2636A smua meas i"() -> (w2805:bool)
                n2866 = Compound Arithmetic op=OR(w2806, w2805, w2804, w2803) -> (w2802:bool)
                n2867 = case shown="True" w2802 {
                  frame False {
                  }
                  frame True {
                    # "close session on 2636A"
                    n2868 = local read "2336A addr"() -> (w2807:refnum<visa-resource-name>)
                    n2869 = VISA Close(VISA resource name=w2807) -> ()  [unwired: 1 in, 1 out]
                  }
                }
              }
            }
          }
          frame #2 {
            n2870 = property on="Step Loop" class="Bool (strict)"() -> ("Value"=w2809:bool)  [unwired: 2 in, 2 out]
            n2871 = case shown="False" w2809 {
              tunnel: w2808 -> [w2812 w2815]
              frame False {
                w2810 = T12."Enabled" ("Disabled")
                n2872 = Enqueue Element(queue=w2812, element="Idle") -> ()  [unwired: 2 in, 3 out]
                n2873 = property on="Sweep Down" class="Bool"("DisabledEnum"=w2810) -> ()  [unwired: 2 in, 2 out]
                n2874 = property on="Sweep Up" class="Bool"("DisabledEnum"=w2810) -> ()  [unwired: 2 in, 2 out]
              }
              frame True {
                n2875 = property on="Sweep Direction" class="Str"() -> ("Value"=w2813:string)  [unwired: 2 in, 2 out]
                n2876 = case shown="\"Sweep Up\"" w2813 {
                  tunnel: w2815 -> [w2816 w2823]
                  frame "Sweep Down", Default {
                    n2877 = stacked-sequence {
                      tunnel: w2816 -> [_ _ w2821]
                      frame #0 {
                        n2878 = property on="Sweep Direction" class="Str"("Value"="Sweep Up" ("Sweep Direction")) -> ()  [unwired: 2 in, 2 out]
                      }
                      frame #1 {
                        n2879 = property on="wait between sweeps(s)" class="DigNum (strict)"() -> ("Value"=w2820:u32)  [unwired: 2 in, 2 out]
                        n2880 = Multiply(x=w2820, y=u32 1000) -> (x*y=w2819:u32)
                        n2881 = Wait (ms)(milliseconds to wait=w2819) -> ()  [unwired: 1 out]
                      }
                      frame #2 {
                        n2882 = Enqueue Element(queue=w2821, element="Step to Next Value") -> ()  [unwired: 2 in, 3 out]
                      }
                    }
                  }
                  frame "Sweep Up" {
                    n2883 = stacked-sequence {
                      tunnel: w2823 -> [_ w2829]
                      frame #0 {
                        n2884 = property on="Table Index" class="DigNum (strict)"() -> ("Value"=w2826:dbl)  [unwired: 2 in, 2 out]
                        n2885 = Increment(x=w2826) -> (x+1=w2825:dbl)
                        n2886 = property on="at field" class="Bool (strict)"("Value"=FALSE ("at field")) -> ()  [unwired: 2 in, 2 out]
                        n2887 = property on="Table Index" class="DigNum (strict)"("Value"=w2825) -> ()  [unwired: 2 in, 2 out]
                        n2888 = property on="Sweep Direction" class="Str"("Value"="Sweep Down" ("Sweep Direction")) -> ()  [unwired: 2 in, 2 out]
                      }
                      frame #1 {
                        n2889 = Enqueue Element(queue=w2829, element="Step to Next Value") -> ()  [unwired: 2 in, 3 out]
                      }
                    }
                  }
                }
                n2890 = property on="Sweep Down" class="Bool"("DisabledEnum"=T12."Disabled and Grayed Out" ("Disabled")) -> ()  [unwired: 2 in, 2 out]
              }
            }
          }
        }
      }
      frame "Ramp To Limit" {
        w3753 = dbl[][] []  # emty array for data
        # "0 = SR830_1_ip\n1 = SR830_1_oop\n2 = SR830_2_ip\n3 = SR830_2_oop\n4 = SR830_3_ip\n5 = SR830_3_oop\n6 = SR830_4_ip \n7 = SR830_4_oop \n8 = SR830_5_ip \n9 = SR830_5_oop \n10 = SR830_6_ip \n11 = SR830_6_oop\n12 = SR830_7_ip \n13 = SR830_7_oop\n14 = SR830_8_ip \n15 = SR830_8_oop\n16 = MFLI_V1\n17 = MFLI_I1\n18 = MFLI_V\n19 = MFLI_I\n20= 2400_1_v \n21= 2400_1_i \n22 = 2400_2_v\n23 = 2400_2_i \n24 = 2400_3_v \n25 = 2400_3_i \n26 = 2182A_1_ch1 \n27 = 2182A_1_ch2 \n28 = 2182A_2_ch1 \n29 = 2182A_2_ch2\n30 = 2182A_3_ch1 \n31 = 2182A_3_ch2 \n32 = 2182A_4_ch1 \n33 = 2182A_4_ch2 \n34 = 2636A_smua_v \n35 = 2636A_smua_i \n36 = 2636A_smub_v \n37 = 2636A_smub_i \n38 = time\n39 = iPS_Field\n40 = iPS_Magnet_T\n41 = iPS__SH_T\n42 = iTC _sample_T\n43 = iTC _VTI_T\n44 = iTC _PT1_T\n45 = iTC _PT2_T\n46 = iTC _VTI_P\n47 = 2461_meas_v\n48= 2461_meas_i\n49= Step_Value\n50= HyperLoop_Step\n51= SuperHyper_Step"
        # "initial time in seconds\nfrom the beginning of month"
        n2891 = stacked-sequence {
          tunnel: [_ _ w4635 _ _] -> w3754
          frame #0 {
            n2892 = local read "2636A smua meas v"() -> (w3763:bool)
            n2893 = local read "2636A smub meas v"() -> (w3761:bool)
            n2894 = local read "2636A smub meas i"() -> (w3760:bool)
            n2895 = local read "2636A smua meas i"() -> (w3762:bool)
            n2896 = property on="sweep" class="RadioBtnsControl (strict)"() -> ("Value"=w3758:T6)  [unwired: 2 in, 2 out]
            n2897 = Compound Arithmetic op=OR(w3763, w3762, w3761, w3760) -> (w3759:bool)
            n2898 = case shown="\"2461\"" w3758 {
              frame "2400_1" {
                # "add label for the first column in the datafile"
                n2899 = stacked-sequence {
                  frame #0 {
                    n2900 = property on="data_caption" class="Str"("Value"="") -> ()  [unwired: 2 in, 2 out]
                    n2901 = property on="Figure_axis" class="Arr (strict)"("Value"=string[] [] ("Figure_axis_string")) -> ()  [unwired: 2 in, 2 out]
                  }
                  frame #1 {
                    w3766 = "V_sweep_2400_1" ("V_sweep")
                    n2902 = Concatenate Strings(w3766, "\t") -> (w3768:string)
                    n2903 = Build Array(w3766) -> (w3767:string[])
                    n2904 = property on="data_caption" class="Str"("Value"=w3768) -> ()  [unwired: 2 in, 2 out]
                    n2905 = property on="Figure_axis" class="Arr (strict)"("Value"=w3767) -> ()  [unwired: 2 in, 2 out]
                  }
                }
              }
              frame "2400_2" {
                n2906 = stacked-sequence {
                  frame #0 {
                    n2907 = property on="data_caption" class="Str"("Value"="") -> ()  [unwired: 2 in, 2 out]
                    n2908 = property on="Figure_axis" class="Arr (strict)"("Value"=string[] [] ("Figure_axis_string")) -> ()  [unwired: 2 in, 2 out]
                  }
                  frame #1 {
                    w3772 = "V_sweep_2400_2" ("V_sweep")
                    n2909 = Build Array(w3772) -> (w3773:string[])
                    n2910 = Concatenate Strings(w3772, "\t") -> (w3775:string)
                    n2911 = property on="Figure_axis" class="Arr (strict)"("Value"=w3773) -> ()  [unwired: 2 in, 2 out]
                    n2912 = property on="data_caption" class="Str"("Value"=w3775) -> ()  [unwired: 2 in, 2 out]
                  }
                }
              }
              frame "2400_3" {
                n2913 = stacked-sequence {
                  frame #0 {
                    n2914 = property on="data_caption" class="Str"("Value"="") -> ()  [unwired: 2 in, 2 out]
                    n2915 = property on="Figure_axis" class="Arr (strict)"("Value"=string[] [] ("Figure_axis_string")) -> ()  [unwired: 2 in, 2 out]
                  }
                  frame #1 {
                    w3778 = "V_sweep_2400_3" ("V_sweep")
                    n2916 = Concatenate Strings(w3778, "\t") -> (w3781:string)
                    n2917 = Build Array(w3778) -> (w3779:string[])
                    n2918 = property on="data_caption" class="Str"("Value"=w3781) -> ()  [unwired: 2 in, 2 out]
                    n2919 = property on="Figure_axis" class="Arr (strict)"("Value"=w3779) -> ()  [unwired: 2 in, 2 out]
                  }
                }
              }
              frame "2636a_smua" {
                n2920 = stacked-sequence {
                  frame #0 {
                    n2921 = property on="data_caption" class="Str"("Value"="") -> ()  [unwired: 2 in, 2 out]
                    n2922 = property on="Figure_axis" class="Arr (strict)"("Value"=string[] [] ("Figure_axis_string")) -> ()  [unwired: 2 in, 2 out]
                  }
                  frame #1 {
                    w3784 = "V_sweep_2636a_smua" ("V_sweep")
                    n2923 = Concatenate Strings(w3784, "\t") -> (w3787:string)
